vi "GetStatus.vi"(8 "error in (no error)":errorcluster, 11 "I2COUSBSim in":refnum<class "I2COUSBSim.lvclass">) -> (0 "error out":errorcluster, 1 "Status":string, 2 "I2CStatus":u8 caption="I2C Status" format="%02x", 3 "I2COUSBSim out":refnum<class "I2COUSBSim.lvclass">)   [LabVIEW 2020, in "I2COUSB.lvlib" / "I2COUSBSim.lvclass"]
doc: "Return the status of the I2C BUS"
uses:
  I2COUSBSim.lvclass
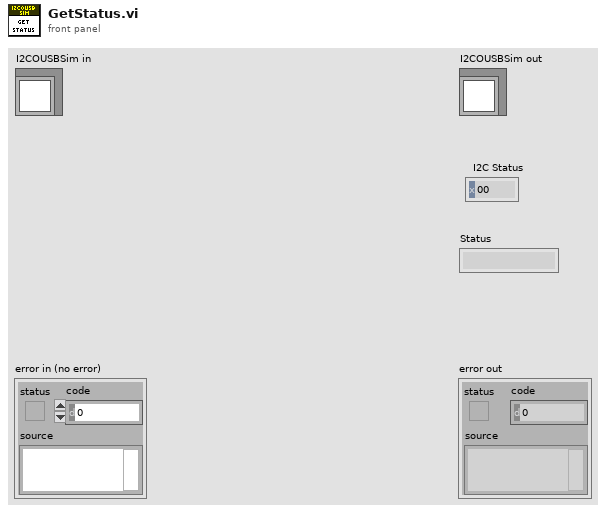
[diagram p1: front panel]
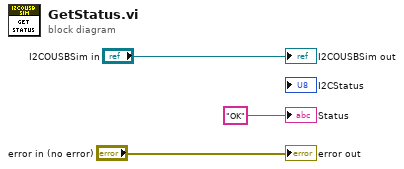
[diagram p0: block diagram]
diagram:
  "error out" <- "error in (no error)"
  "I2COUSBSim out" <- "I2COUSBSim in"
  "Status" <- "OK" ("Status")
